vi "LvMPDC_SUB_ParseReplyString_MusicInfo.vi"(10 "status reply string":string="file: musiclibrary/Konan_2/Everlasting.mp3\nLast-Modified: 2015-02-13T13:27:50Z\nTime: 221\nArtist: B'z\nTitle: Everlasting\nAlbum: KONAN BEST 2\nTrack: 1/15\nGenre: Jpop\n") -> (2 "MusicInfo":T1)   [LabVIEW 2012]
uses:
  LvMPDC_Typdef_MusicInfo.ctl
panel:
  # "file: musiclibrary/Konan_2/Everlasting.mp3\nLast-Modified: 2015-02-13T13:27:50Z\nTime: 221\nArtist: B'z\nTitle: Everlasting\nAlbum: KONAN BEST 2\nTrack: 1/15\nGenre: Jpop"
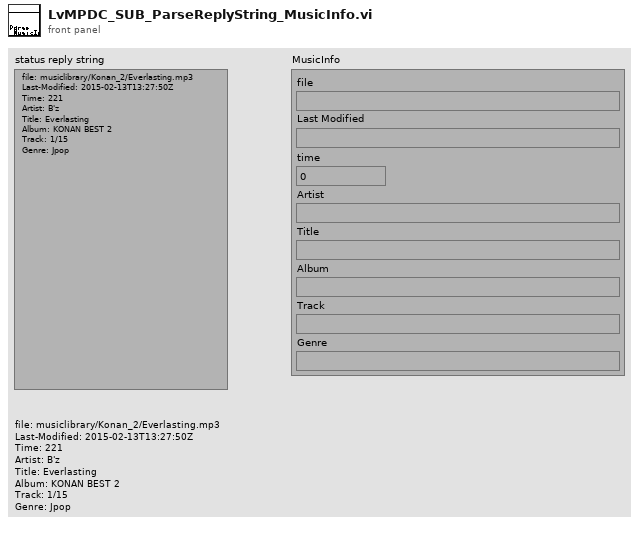
[diagram p1: front panel]
types:
  T1 = typedef "LvMPDC_Typdef_MusicInfo.ctl" = cluster{"file":string, "Last Modified":string, "time":dbl, "Artist":string, "Title":string, "Album":string, "Track":string, "Genre":string}
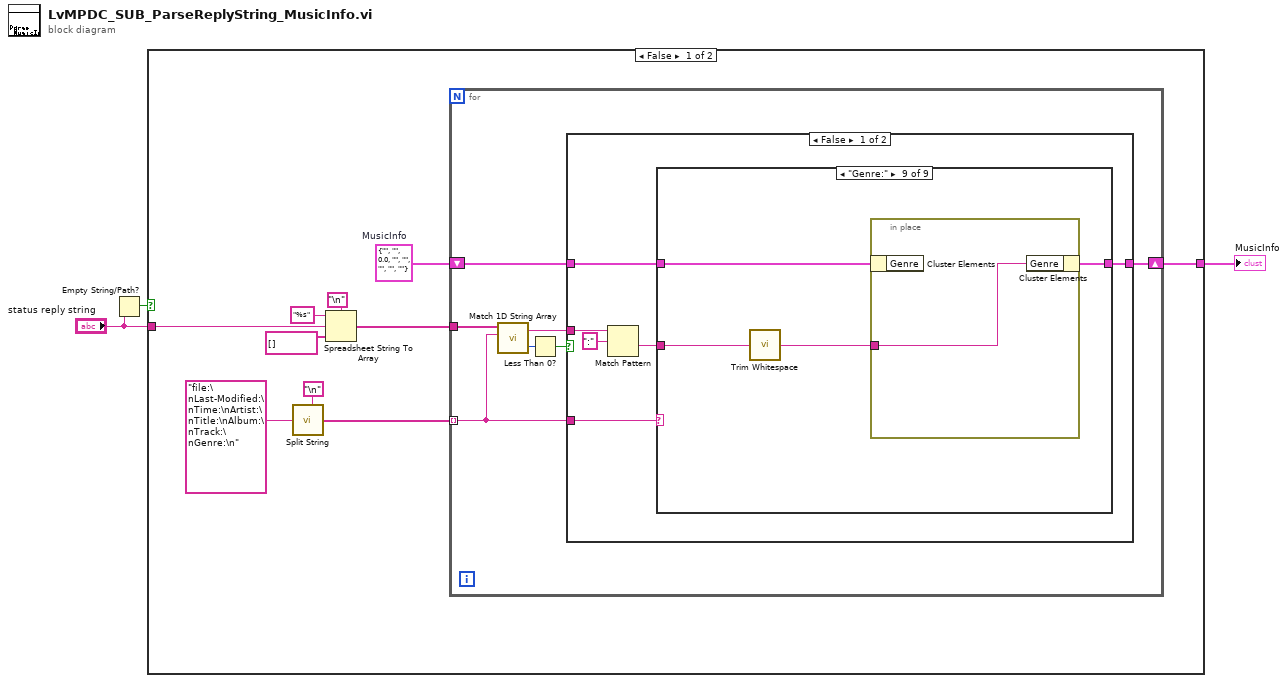
[diagram p0: block diagram]
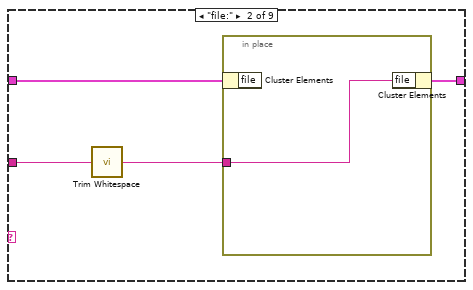
[diagram p3: hidden frame]
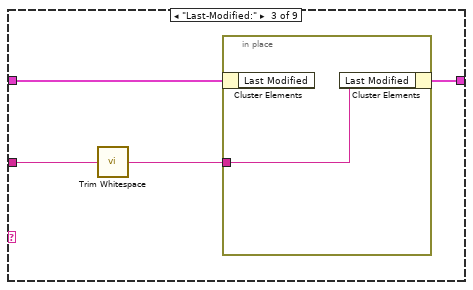
[diagram p4: hidden frame]
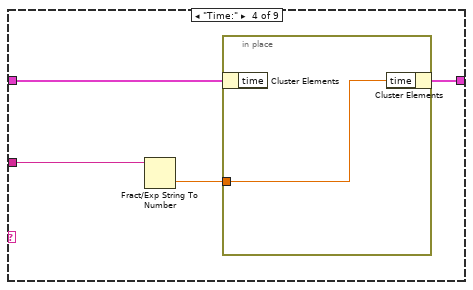
[diagram p5: hidden frame]
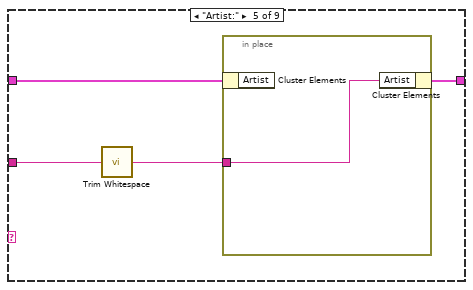
[diagram p6: hidden frame]
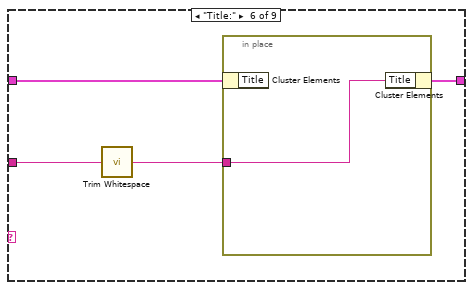
[diagram p7: hidden frame]
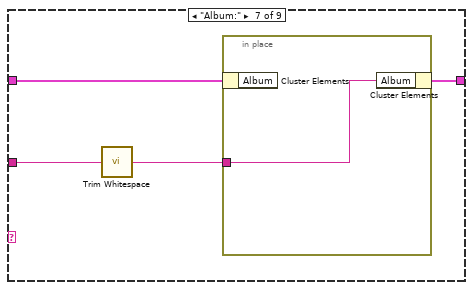
[diagram p8: hidden frame]
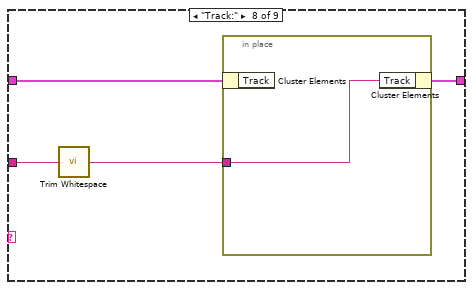
[diagram p9: hidden frame]
diagram:
  n1 = Empty String/Path?(string/path="status reply string") -> (empty?=w1:bool)
  n2 = case shown="FALSE" w1 {
    tunnel: "status reply string" -> [w10 _]
    tunnel: [w6 _] -> w3
    frame False {
      w4 = T1 {"file"="", "Last Modified"="", "time"=0.0, "Artist"="", "Title"="", "Album"="", "Track"="", "Genre"=""}  # MusicInfo
      n3 = call <vilib>:"Split String.vi"("Split Pattern"="\n", "Input String"="file:\nLast-Modified:\nTime:\nArtist:\nTitle:\nAlbum:\nTrack:\nGenre:\n") -> ("Split String"=w7:string[])  [unwired: 5 in]
      n4 = Spreadsheet String To Array(delimiter (Tab)="\n", format string="%s" ("形式文字列"), spreadsheet string=w10, array type (2D Dbl)=string[] []) -> (array=w9:string[])
      n5 = for {
        tunnel: w9 -> [w20]
        tunnel: w7 -> [w19] mode=indexing
        shift-right: [w14] -> w6
        shift-left: w4 -> [w15]
        n6 = call <vilib>:"Match 1D String Array.vi"("Pattern"=w19, "Strings"=w20) -> ("index of element"=w18:i32, "Match"=w17:string)  [unwired: 2 in]
        n7 = Less Than 0?(x=w18) -> (x < 0?=w16:bool)
        n8 = case shown="FALSE" w16 {
          tunnel: w19 -> [w26 _]
          tunnel: w17 -> [w22 _]
          tunnel: w15 -> [w25 w68]
          tunnel: [w24 w68] -> w14
          frame False {
            n9 = Match Pattern(string=w22, regular expression=":" ("正規表現")) -> (after substring=w21:string)  [unwired: 1 in, 3 out]
            n10 = case shown="\"Genre:\"" w26 {
              tunnel: w25 -> [w27 w31 w36 w41 w46 w51 w56 w61 w66]
              tunnel: [w27 w30 w35 w40 w45 w50 w55 w60 w65] -> w24
              tunnel: w21 -> [_ w29 w34 w39 w44 w49 w54 w59 w64]
              frame Default {
              }
              frame "file:" {
                n11 = call <vilib>:"Trim Whitespace.vi"("string"=w29) -> ("trimmed string"=w28:string)  [unwired: 1 in]
                n12 = in-place {
                  in-place-border: w28 -> [w32]
                  n13 = in-place-cluster #1(w31) -> ()  [unwired: 1 out]
                  n14 = in-place-cluster #1("file"=w32) -> (w30:T1)
                }
              }
              frame "Last-Modified:" {
                n15 = call <vilib>:"Trim Whitespace.vi"("string"=w34) -> ("trimmed string"=w33:string)  [unwired: 1 in]
                n16 = in-place {
                  in-place-border: w33 -> [w37]
                  n17 = in-place-cluster #2(w36) -> ()  [unwired: 1 out]
                  n18 = in-place-cluster #2("Last Modified"=w37) -> (w35:T1)
                }
              }
              frame "Time:" {
                n19 = Fract/Exp String To Number(string=w39) -> (number=w38:dbl)  [unwired: 3 in, 1 out]
                n20 = in-place {
                  in-place-border: w38 -> [w42]
                  n21 = in-place-cluster #3(w41) -> ()  [unwired: 1 out]
                  n22 = in-place-cluster #3("time"=w42) -> (w40:T1)
                }
              }
              frame "Artist:" {
                n23 = call <vilib>:"Trim Whitespace.vi"("string"=w44) -> ("trimmed string"=w43:string)  [unwired: 1 in]
                n24 = in-place {
                  in-place-border: w43 -> [w47]
                  n25 = in-place-cluster #4(w46) -> ()  [unwired: 1 out]
                  n26 = in-place-cluster #4("Artist"=w47) -> (w45:T1)
                }
              }
              frame "Title:" {
                n27 = call <vilib>:"Trim Whitespace.vi"("string"=w49) -> ("trimmed string"=w48:string)  [unwired: 1 in]
                n28 = in-place {
                  in-place-border: w48 -> [w52]
                  n29 = in-place-cluster #5(w51) -> ()  [unwired: 1 out]
                  n30 = in-place-cluster #5("Title"=w52) -> (w50:T1)
                }
              }
              frame "Album:" {
                n31 = call <vilib>:"Trim Whitespace.vi"("string"=w54) -> ("trimmed string"=w53:string)  [unwired: 1 in]
                n32 = in-place {
                  in-place-border: w53 -> [w57]
                  n33 = in-place-cluster #6(w56) -> ()  [unwired: 1 out]
                  n34 = in-place-cluster #6("Album"=w57) -> (w55:T1)
                }
              }
              frame "Track:" {
                n35 = call <vilib>:"Trim Whitespace.vi"("string"=w59) -> ("trimmed string"=w58:string)  [unwired: 1 in]
                n36 = in-place {
                  in-place-border: w58 -> [w62]
                  n37 = in-place-cluster #7(w61) -> ()  [unwired: 1 out]
                  n38 = in-place-cluster #7("Track"=w62) -> (w60:T1)
                }
              }
              frame "Genre:" {
                n39 = call <vilib>:"Trim Whitespace.vi"("string"=w64) -> ("trimmed string"=w63:string)  [unwired: 1 in]
                n40 = in-place {
                  in-place-border: w63 -> [w67]
                  n41 = in-place-cluster #8(w66) -> ()  [unwired: 1 out]
                  n42 = in-place-cluster #8("Genre"=w67) -> (w65:T1)
                }
              }
            }
          }
          frame True {
          }
        }
      }
    }
    frame True {
    }
  }
  "MusicInfo" <- w3
